vi "Crop Roi.vi"(10 "Roi":T1, 11 "Table Roi In":i32[][](array[numeric])) -> (3 "Table Roi Out":i32[][](array[numeric]))   [LabVIEW 2023]
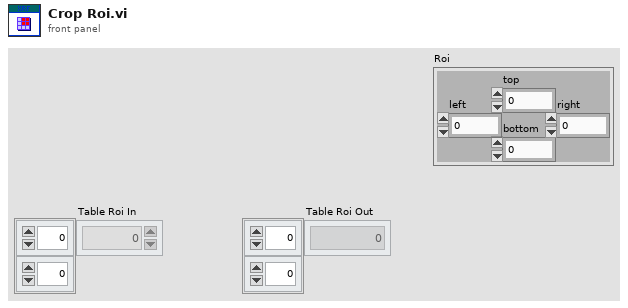
[diagram p1: front panel]
types:
  T1 = cluster{"left":i16, "top":i16, "right":i16, "bottom":i16}
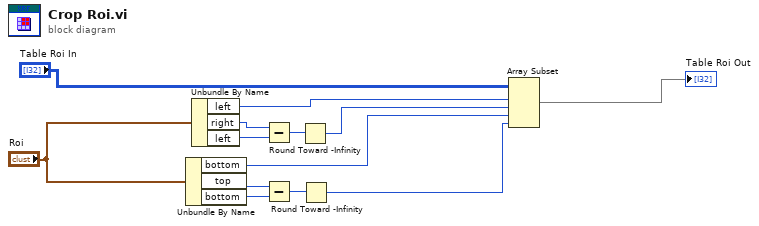
[diagram p0: block diagram]
diagram:
  n1 = Unbundle By Name("Roi") -> ("bottom"=w5:i16, "top"=w8:i16, "bottom"=w9:i16)
  n2 = Unbundle By Name("Roi") -> ("left"=w7:i16, "right"=w13:i16, "left"=w12:i16)
  n3 = Subtract(x=w13, y=w12) -> (x-y=w11:i16)
  n4 = Subtract(x=w8, y=w9) -> (x-y=w10:i16)
  n5 = Round Toward -Infinity(1:w11) -> (0:w6:i16)
  n6 = Round Toward -Infinity(1:w10) -> (0:w4:i16)
  n7 = Array Subset(array="Table Roi In", index (row)=w7, length (row)=w6, index (col)=w5, length (col)=w4) -> (→"Table Roi Out":i32[][])
